vi "AlliGator Read set File.vi"(8 "Error In":errorcluster, 11 "Image Folder Path":path) -> (0 "Error Out":errorcluster, 1 "Metadata":T1 {"Date" format="%<%x %.3X>T"}, 2 "File Info String":string, 3 ".set File dup":path, 5 "File info":variant)   [LabVIEW 2021, in "AlliGator Files.lvlib"]
doc: "Tries to extract FLI dataset metadata corresponding to one of LaVision formats."
uses:
  AlliGator Files.lvlib
  AlliGator RecSettings Metadata.ctl
  AlliGator RecSettings Metadata Field.ctl
  <vilib>/Utility/error.llb/whitespace.ctl
  Time/PicoStart Date.ctl
  Strings/Strings.lvlib
  Time/Time.lvlib
panel:
  out "Time (s)":dbl
  # "see the AlliGator License on the block diagram (Ctrl+E or Window:Show Block Diagram)"
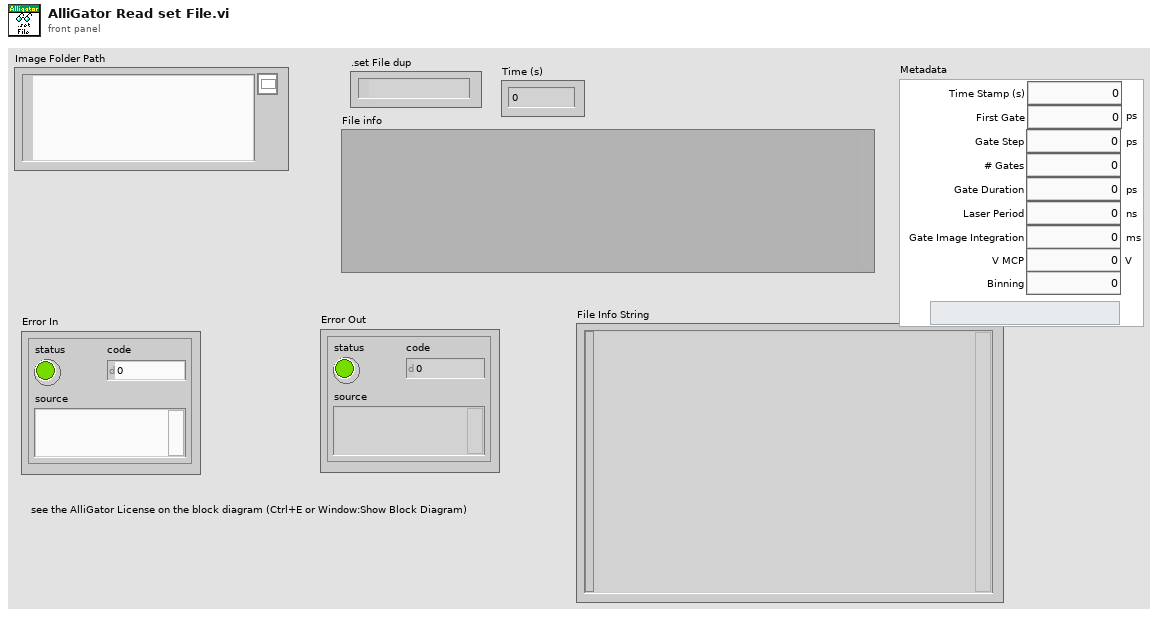
[diagram p1: front panel]
types:
  T1 = typedef "AlliGator Files.lvlib/AlliGator RecSettings Metadata.ctl" = cluster{"Time Stamp (s)":dbl, "First Gate":dbl[unit], "Gate Step":dbl[unit], "# Gates":i32, "Gate Duration":dbl[unit], "Laser Period":dbl[unit], "Gate Image Integration":dbl[unit], "Date":timestamp, "V MCP":dbl[unit], "Binning":dbl}
  T2 = typedef "AlliGator Files.lvlib/AlliGator RecSettings Metadata Field.ctl" = enum16{"Time", "Gate Start", "Gate Step", "# Gates", "Gate Duration", "Laser Period", "Gate Image Integration", "MCP Voltage", "Binning"}
  T3 = typedef "Time.lvlib/PicoStart Date.ctl" = cluster{"Day in Week":string, "Month":string, "Day":i32, "Hours":i32, "Minutes":i32, "Seconds":i32, "Year":i32}
  T4 = typedef "whitespace.ctl" = u16
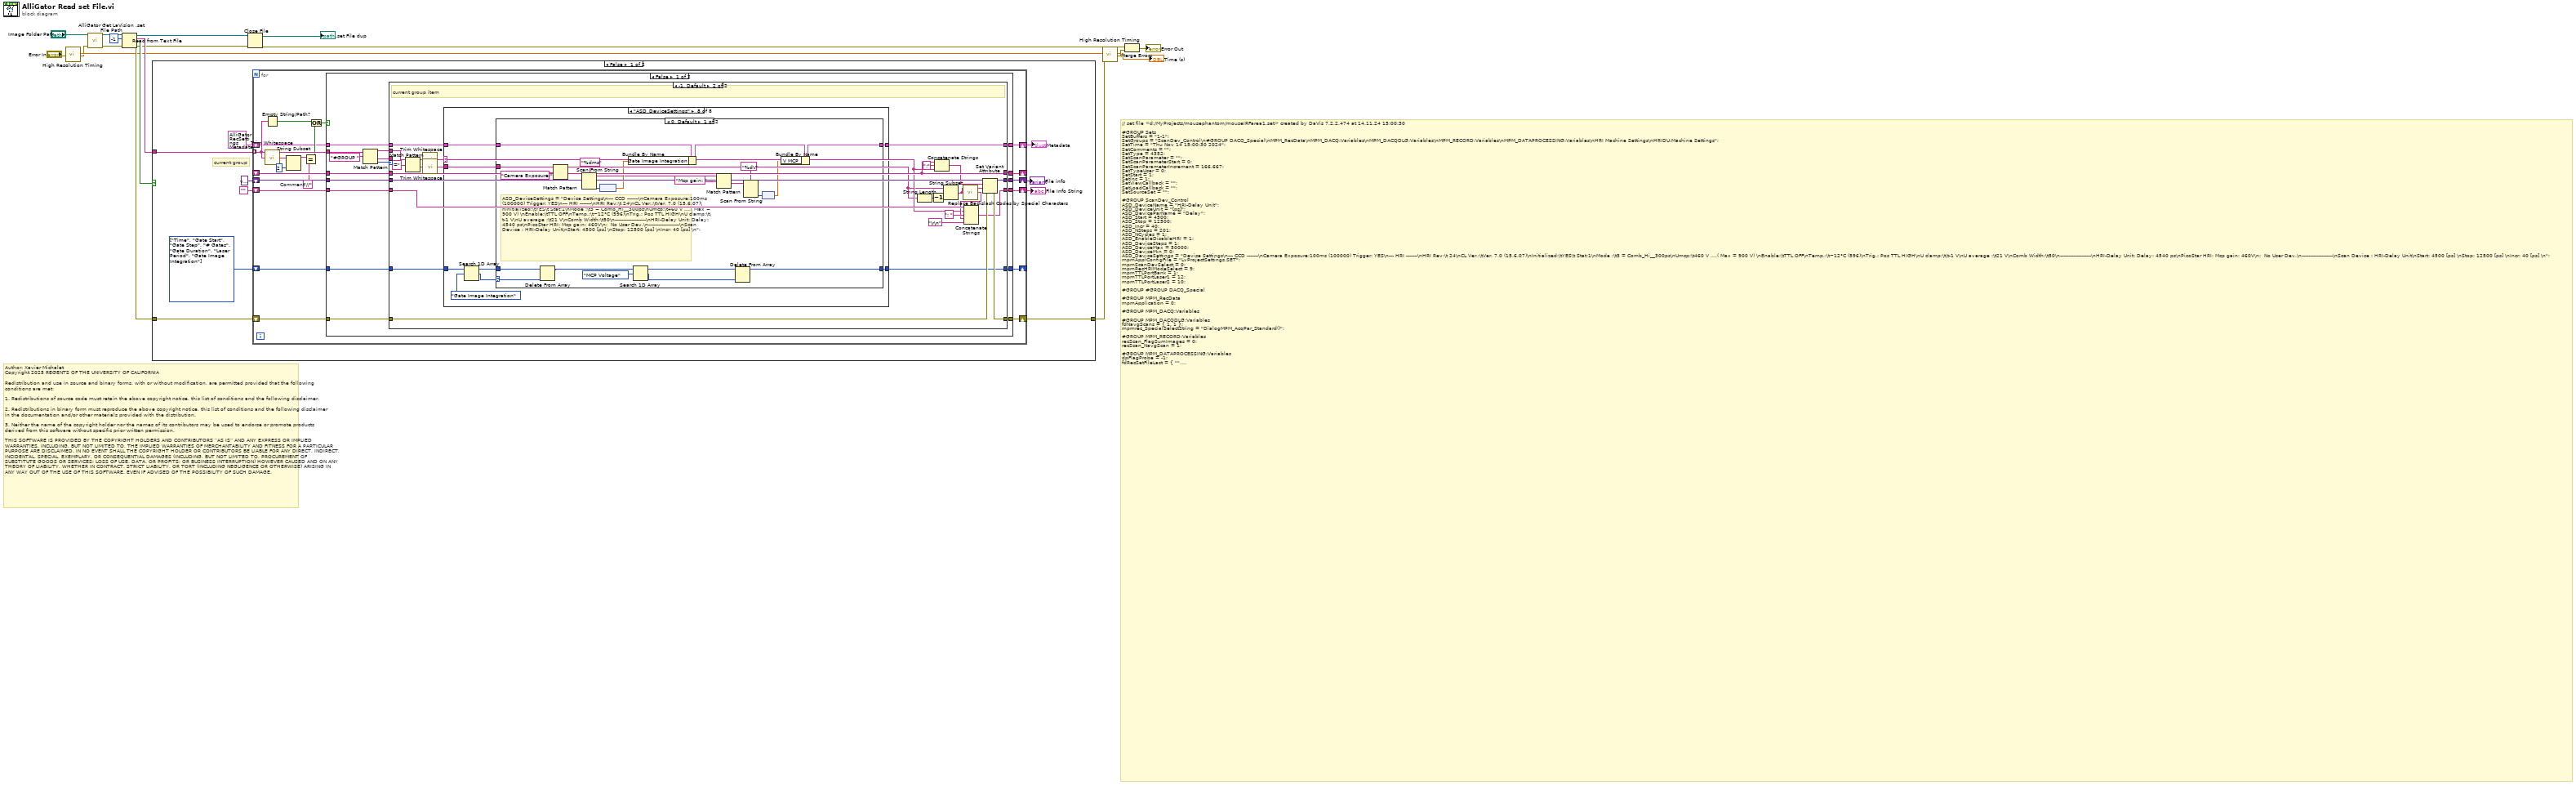
[diagram p0: block diagram]
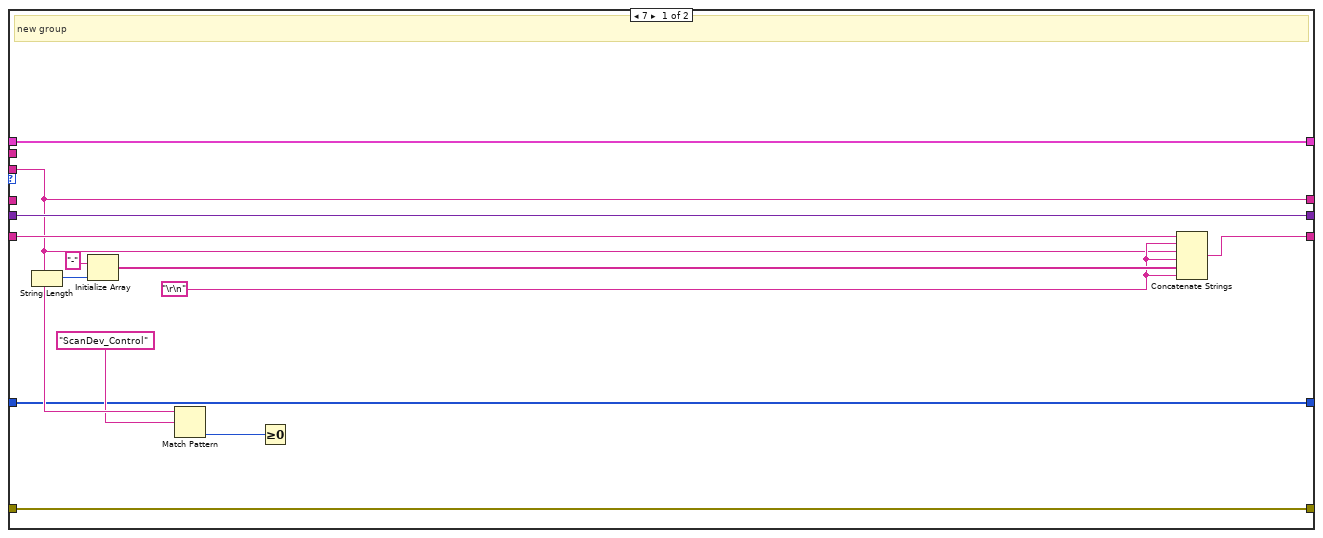
[diagram p2: hidden frame]
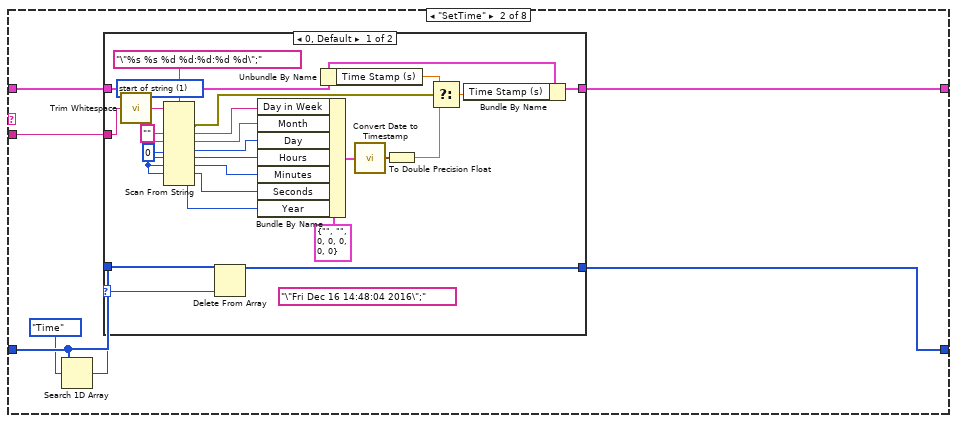
[diagram p4: hidden frame]
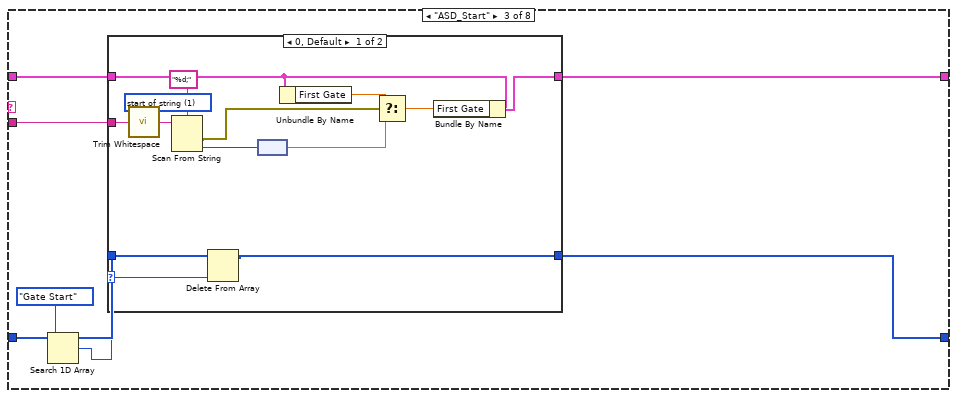
[diagram p6: hidden frame]
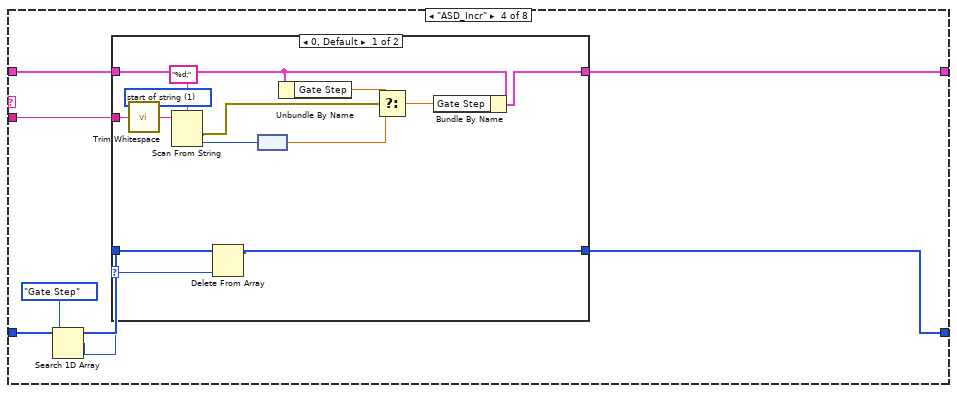
[diagram p8: hidden frame]
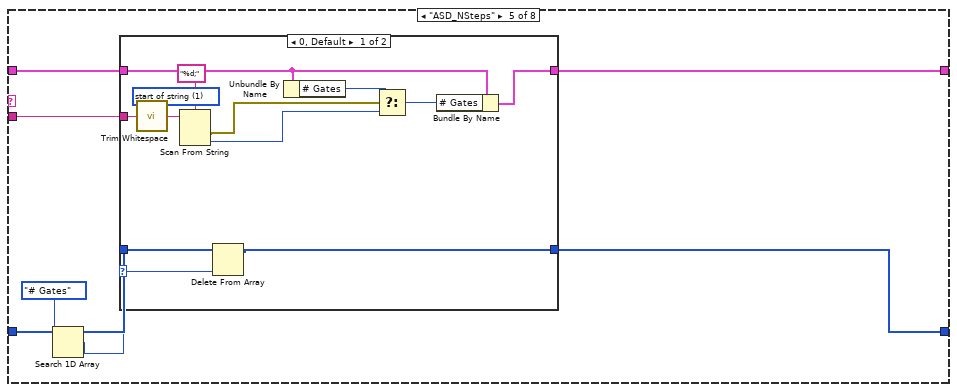
[diagram p10: hidden frame]
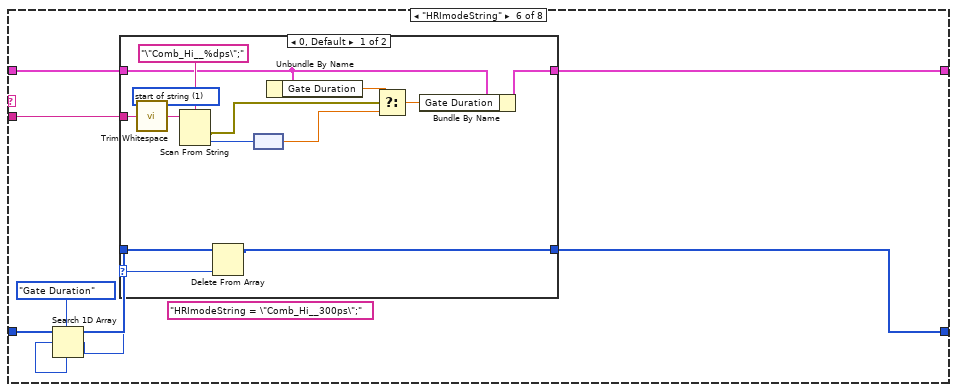
[diagram p12: hidden frame]
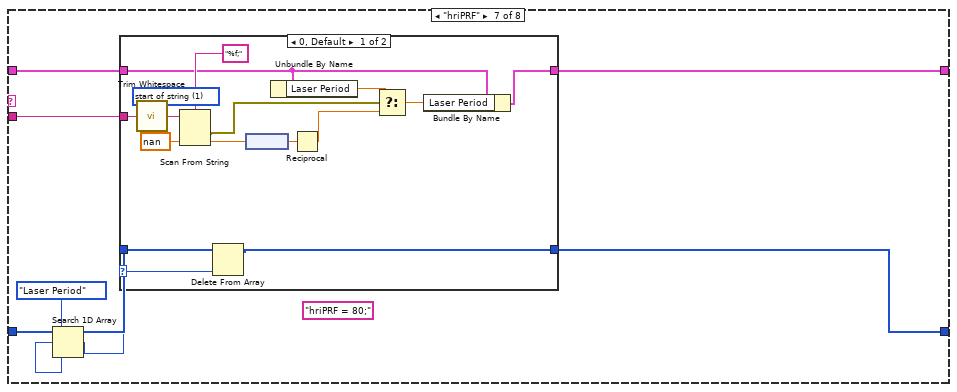
[diagram p14: hidden frame]
diagram:
  # "// set file <d:/MyProjects/mousephantom/mouseIRFarea1.set> created by DaVis 7.2.2.474 at 14.11.24 15:00:30\n\n#GROUP Sets\nSetBuffers = \"1-1\";  \nSetGroups = \"ScanDev_Control\\n#GROUP DACQ_Special\\nMPM_RecData\\nMPM_DACQ:Variables\\nMPM_DACQDLG:Variables\\nMPM_RECORD:Variables\\nMPM_DATAPROCESSING:Variables\\nHRI Machine Settings\\nHRIDU:Machine Settings\";\nSetTime = \"Thu Nov 14 15:00:30 2024\";\nSetComments = \"\";\nSetType = 4352;\nSetScanParameter = \"\";\nSetScanParameterStart = 0;\nSetScanParameterIncrement = 166.667;\nSetTypeUser = 0;\nSetStart = 1;\nSetInc = 1;\nSetViewCallback = \"\";\nSetLoadCallback = \"\";\nSetSourceSet = \"\";\n\n#GROUP ScanDev_Control\nASD_DeviceName = \"HRI-Delay Unit\";\nASD_DeviceUnit = \"[ps]\";\nASD_DeviceParName = \"Delay\";\nASD_Start = 4500;\nASD_Stop = 12500;\nASD_Incr = 40;\nASD_NSteps = 201;\nASD_NCycles = 1;\nASD_EnableDisableHRI = 1;\nASD_DeviceSteps = 1;\nASD_DeviceMax = 50000;\nASD_DeviceMin = 0;\nASD_DeviceSettings = \"Device Settings\\n--- CCD -------\\nCamera Exposure:100ms (100000) Trigger: YES\\n--- HRI -------\\nHRI Rev:\\t 24\\nCL Ver.:\\tVer. 7.0 (15.6.07)\\nInitialized:\\tYES\\t Stat:1\\nMode :\\t3 = Comb_Hi__300ps\\nUmcp:\\t460 V ....( Max = 900 V) \\nEnable:\\tTTL OFF\\nTemp.:\\t~12°C (596)\\nTrig.: Pos TTL HIGH\\nU clamp:\\t\\t-1 V\\nU average :\\t21 V\\nComb Width:\\t50\\n-------------------\\nHRI-Delay Unit: Delay: 4540 ps\\nPicoStar HRI: Mcp gain: 460V\\n:  No User Dev.\\n-------------------\\nScan Device : HRI-Delay Unit\\nStart: 4500 [ps] \\nStop: 12500 [ps] \\nIncr: 40 [ps] \\n\";\nmpmApplConfigFile = \"LvProjectSettings.SET\";\nmpmScanDevSelect = 0;\nmpmRecHRIModeSelect = 9;\nmpmTTLPortBank = 1;\nmpmTTLPortLaser1 = 12;\nmpmTTLPortLaser2 = 10;\n\n#GROUP #GROUP DACQ_Special\n\n#GROUP MPM_RecData\nmpmApplication = 0;\n\n#GROUP MPM_DACQ:Variables\n\n#GROUP MPM_DACQDLG:Variables\nfdNavgScans = { 1, 1 };\nmpmrec_SpecialSelectString = \"DialogMPM_AcqPar_Standard()\";\n\n#GROUP MPM_RECORD:Variables\nrecScan_FlagSumImages = 0;\nrecScan_NavgScan = 1;\n\n#GROUP MPM_DATAPROCESSING:Variables\ndpFlagProbe = -1;\nfdRecSetFileLast = { \"\", \"\" };\nmpmFlag_UseFitDLL = 1;\nflimfd_Freq = 80;\nflimFlagShowTrace = 1;\n\n#GROUP HRI Machine Settings\nhriPRF = 80;\nHRIType = 0;\nHRIMode = 3;\nHRIGain = 430;\nHRITrig_Edge = 1;\nHRITrig_Typ = 0;\nHRITrig_Level = 0;\nHRITrig_Term = 0;\nHRIThresh = 0.4;\nHRIClamp = -1;\nHRIAverage = 21;\nHRICombWidth = 50;\nHRIRFgain = 60;\nHRIRFgainIncr = 10;\nhriTempString = \"~12°C (596)\";\nHRIRateTune = 3;\nHRImodeString = \"Comb_Hi__300ps\";\nHRIGOIMode = 0;\n\n#GROUP HRIDU:Machine Settings\nhridu_40MHz_copy = 0;\nhridu_Trg_Coupling_copy = 1;\nhridu_Trg_Term_copy = 1;\nhridu_Trg_Edge_copy = 1;\nhridu_Trg_Attenuator_copy = 0;\nhridu_Trg_Thresh_copy = 102;\nhridu_Delay_copy = 7740;\nhridu_ScanDelayStart_copy = 0;\nhridu_ScanDelayStop_copy = 12000;\nhridu_ScanDelayIncr_copy = 40;"
  # "Author: Xavier Michalet\nCopyright 2025 REGENTS OF THE UNIVERSITY OF CALIFORNIA\n\nRedistribution and use in source and binary forms, with or without modification, are permitted provided that the following conditions are met:\n\n1. Redistributions of source code must retain the above copyright notice, this list of conditions and the following disclaimer.\n\n2. Redistributions in binary form must reproduce the above copyright notice, this list of conditions and the following disclaimer in the documentation and/or other materials provided with the distribution.\n\n3. Neither the name of the copyright holder nor the names of its contributors may be used to endorse or promote products derived from this software without specific prior written permission.\n\nTHIS SOFTWARE IS PROVIDED BY THE COPYRIGHT HOLDERS AND CONTRIBUTORS “AS IS” AND ANY EXPRESS OR IMPLIED WARRANTIES, INCLUDING, BUT NOT LIMITED TO, THE IMPLIED WARRANTIES OF MERCHANTABILITY AND FITNESS FOR A PARTICULAR PURPOSE ARE DISCLAIMED. IN NO EVENT SHALL THE COPYRIGHT HOLDER OR CONTRIBUTORS BE LIABLE FOR ANY DIRECT, INDIRECT, INCIDENTAL, SPECIAL, EXEMPLARY, OR CONSEQUENTIAL DAMAGES (INCLUDING, BUT NOT LIMITED TO, PROCUREMENT OF SUBSTITUTE GOODS OR SERVICES; LOSS OF USE, DATA, OR PROFITS; OR BUSINESS INTERRUPTION) HOWEVER CAUSED AND ON ANY THEORY OF LIABILITY, WHETHER IN CONTRACT, STRICT LIABILITY, OR TORT (INCLUDING NEGLIGENCE OR OTHERWISE) ARISING IN ANY WAY OUT OF THE USE OF THIS SOFTWARE, EVEN IF ADVISED OF THE POSSIBILITY OF SUCH DAMAGE."
  n1 = call "High Resolution Timing.vi"("Error In"="Error In") -> ("elapsed (relative) seconds"=w7:dbl, "Error Out"=w2:errorcluster)  [unwired: 16 in, 1 out]
  n2 = call "AlliGator Get LaVision .set File Path.vi"("Error In"=w2, "Gate Image Folder Path"="Image Folder Path") -> ("Error Out"=w1:errorcluster, ".set File Path"=w4:path)  [unwired: 8 in]
  n3 = Read from Text File(file (use dialog)=w4, count=-1, error in=w1) -> (refnum out=w16:refnum<file>, text=w14:string[], cancelled=w13:bool, error out=w11:errorcluster)  [unwired: 1 in]
  n4 = case shown="False" w13 {
    tunnel: w14 -> [w27 _]
    tunnel: w11 -> [w24 w291]
    tunnel: [w23 w291] -> w10
    frame False {
      w19 = T2[] [enum."Time", enum."Gate Start", enum."Gate Step", enum."# Gates", enum."Gate Duration", enum."Laser Period", enum."Gate Image Integration"] items=["Time", "Gate Start", "Gate Step", "# Gates", "Gate Duration", "Laser Period", "Gate Image Integration", "MCP Voltage", "Binning"] ("Array")
      # "current group"
      n5 = for {
        tunnel: w27 -> [w41] mode=indexing
        shift-right: [w45] -> _
        shift-left: _ -> [w46]
        shift-right: [w44] -> w25
        shift-left: variant -> [w43]
        shift-right: [w34] -> w23
        shift-left: w24 -> [w35]
        shift-right: [w32] -> w21
        shift-left: "" -> [w33]
        shift-right: [w31] -> w20
        shift-left: T1 {"Time Stamp (s)"=nan, "First Gate"=nan, "Gate Step"=nan, "# Gates"=0, "Gate Duration"=nan, "Laser Period"=nan, "Gate Image Integration"=nan, "Date"=timestamp(0 s since 1904-01-01), "V MCP"=nan, "Binning"=nan} ("Metadata") -> [w30]
        shift-right: [w28] -> _
        shift-left: w19 -> [w29]
        w37 = "//"  # Comment
        n6 = call <vilib>:"Trim Whitespace.vi"("string"=w41) -> ("trimmed string"=w40:string)  [unwired: 1 in]
        n7 = Empty String/Path?(string/path=w41) -> (empty?=w47:bool)
        n8 = String Subset(string=w40, length (rest)=2 ("length (rest)")) -> (substring=w38:string)  [unwired: 1 in]
        n9 = Equal?(x=w38, y=w37) -> (x = y?=w36:bool)
        n10 = Or(x=w47, y=w36) -> (x .or. y?=w42:bool)
        n11 = case shown="False" w42 {
          tunnel: w41 -> [w63 _]
          tunnel: w46 -> [w57 w290]
          tunnel: [w60 w290] -> w45
          tunnel: [w59 w289] -> w44
          tunnel: w43 -> [w58 w289]
          tunnel: w35 -> [w55 w288]
          tunnel: [w54 w288] -> w34
          tunnel: w33 -> [w53 w287]
          tunnel: [w52 w287] -> w32
          tunnel: [w51 w286] -> w31
          tunnel: w30 -> [w50 w286]
          tunnel: w29 -> [w49 w285]
          tunnel: [w48 w285] -> w28
          frame False {
            n12 = Match Pattern(string=w63, regular expression="#GROUP ") -> (before substring=w56:string, after substring=w61:string, offset past match=w62:i32)  [unwired: 1 in, 1 out]
            n13 = case shown="-1, Default" w62 {
              tunnel: w61 -> [w68 _]
              tunnel: [w68 w96] -> w60
              tunnel: [w77 w100] -> w59
              tunnel: w58 -> [w77 w99]
              tunnel: w57 -> [_ w96]
              tunnel: w56 -> [_ w94]
              tunnel: w55 -> [w76 w93]
              tunnel: [w76 w92] -> w54
              tunnel: w53 -> [w75 w91]
              tunnel: [w71 w87] -> w52
              tunnel: [w69 w81] -> w51
              tunnel: w50 -> [w69 w80]
              tunnel: w49 -> [w65 w79]
              tunnel: [w65 w78] -> w48
              frame 7 {
                w70 = "\r\n"
                # "new group"
                n14 = String Length(string=w68) -> (length=w74:i32)
                n15 = Initialize Array("-", w74) -> (w72:string[])
                n16 = Match Pattern(string=w68, regular expression="ScanDev_Control") -> (offset past match=w66:i32)  [unwired: 1 in, 3 out]
                n17 = Greater Or Equal To 0?(x=w66) -> ()  [unwired: 1 out]
                n18 = Concatenate Strings(w75, w70, w68, w70, w72, w70) -> (w71:string)
              }
              frame -1, Default {
                # "current group item"
                n19 = Match Pattern(string=w94, regular expression="=") -> (before substring=w101:string, after substring=w83:string)  [unwired: 1 in, 2 out]
                n20 = call <vilib>:"Trim Whitespace.vi"("string"=w101) -> ("trimmed string"=w84:string)  [unwired: 1 in]
                n21 = call <vilib>:"Trim Whitespace.vi"("string"=w83) -> ("trimmed string"=w82:string)  [unwired: 1 in]
                n22 = case shown="\"ASD_DeviceSettings\"" w84 {
                  tunnel: w82 -> [_ w111 w144 w167 w190 w212 w235 w260]
                  tunnel: [w104 w109 w145 w168 w191 w213 w236 w261] -> w81
                  tunnel: w80 -> [w104 w110 w143 w166 w189 w211 w234 w259]
                  tunnel: w79 -> [w103 w107 w141 w164 w187 w209 w232 w257]
                  tunnel: [w103 w108 w139 w162 w185 w207 w230 w255] -> w78
                  frame "", Default {
                  }
                  frame "SetTime" {
                    n23 = Search 1D Array(1D array=w107, element=AlliGator_RecSettings_Metadata_Field."Time" ("Metadata Field")) -> (index of element=w105:i32)  [unwired: 1 in]
                    n24 = case shown="0, Default" w105 {
                      selector: w105 -> [w112 _]
                      tunnel: w111 -> [w117 _]
                      tunnel: w110 -> [w116 w138]
                      tunnel: [w115 w138] -> w109
                      tunnel: [w114 w137] -> w108
                      tunnel: w107 -> [w113 w137]
                      frame 0, Default {
                        (unwired) "\"Fri Dec 16 14:48:04 2016\";"
                        w123 = 0 ("default value 3")
                        w124 = "" ("default value 1")
                        w135 = T4 1 items=["both", "start of string", "end of string"] ("location (both)")
                        n25 = call <vilib>:"Trim Whitespace.vi"("string"=w117, "location (both)"=w135) -> ("trimmed string"=w126:string)
                        n26 = Scan From String(format string="\"%s %s %d %d:%d:%d %d\";", input string=w126, default 1=w124, default 2=w124, default 3=w123, default 4=w123, default 5=w123, default 6=w123) -> (error out=w122:errorcluster, output 1=w134:string, output 2=w133:string, output 3=w132:i32, output 4=w131:i32, output 5=w130:i32, output 6=w129:i32, output 7=w118:i32)  [unwired: 3 in, 2 out]
                        n27 = Delete From Array(array=w113, index=w112) -> (array with subset deleted=w114:T2[])  [unwired: 1 in, 1 out]
                        n28 = Bundle By Name(cluster=T3 {"Day in Week"="", "Month"="", "Day"=0, "Hours"=0, "Minutes"=0, "Seconds"=0, "Year"=0}, "Day in Week"=w134, "Month"=w133, "Day"=w132, "Hours"=w131, "Minutes"=w130, "Seconds"=w129, "Year"=w118) -> (w128:T3)
                        n29 = Unbundle By Name(w116) -> ("Time Stamp (s)"=w119:dbl)
                        n30 = call "Convert Date to Timestamp.vi"("Date"=w128) -> ("Time Stamp"=w136:timestamp)  [unwired: 8 in]
                        n31 = To Double Precision Float(number=w136) -> (double precision float=w120:dbl)
                        n32 = Select(t=w119, s=w122, f=w120) -> (s? t:f=w121:dbl)
                        n33 = Bundle By Name(cluster=w116, "Time Stamp (s)"=w121) -> (w115:T1)
                      }
                      frame -1 {
                      }
                    }
                  }
                  frame "ASD_Start" {
                    n34 = Search 1D Array(1D array=w141, element=AlliGator_RecSettings_Metadata_Field."Gate Start" ("Metadata Field")) -> (index of element=w140:i32)  [unwired: 1 in]
                    n35 = case shown="0, Default" w140 {
                      selector: w140 -> [w147 _]
                      tunnel: [w159 w161] -> w145
                      tunnel: w144 -> [w155 _]
                      tunnel: w143 -> [w152 w161]
                      tunnel: w141 -> [w148 w160]
                      tunnel: [w146 w160] -> w139
                      frame 0, Default {
                        w158 = T4 1 items=["both", "start of string", "end of string"] ("location (both)")
                        n36 = call <vilib>:"Trim Whitespace.vi"("string"=w155, "location (both)"=w158) -> ("trimmed string"=w157:string)
                        n37 = Scan From String(format string="%d;", input string=w157) -> (error out=w154:errorcluster, output 1=w150:i32)  [unwired: 3 in, 2 out]
                        n38 = Delete From Array(array=w148, index=w147) -> (array with subset deleted=w146:T2[])  [unwired: 1 in, 1 out]
                        n39 = node(w150) -> (w149:dbl[unit])
                        n40 = Unbundle By Name(w152) -> ("First Gate"=w151:dbl[unit])
                        n41 = Select(t=w151, s=w154, f=w149) -> (s? t:f=w153:dbl[unit])
                        n42 = Bundle By Name(cluster=w152, "First Gate"=w153) -> (w159:T1)
                      }
                      frame -1 {
                      }
                    }
                  }
                  frame "ASD_Incr" {
                    n43 = Search 1D Array(1D array=w164, element=AlliGator_RecSettings_Metadata_Field."Gate Step" ("Metadata Field")) -> (index of element=w163:i32)  [unwired: 1 in]
                    n44 = case shown="0, Default" w163 {
                      selector: w163 -> [w170 _]
                      tunnel: [w182 w184] -> w168
                      tunnel: w167 -> [w178 _]
                      tunnel: w166 -> [w175 w184]
                      tunnel: w164 -> [w171 w183]
                      tunnel: [w169 w183] -> w162
                      frame 0, Default {
                        w181 = T4 1 items=["both", "start of string", "end of string"] ("location (both)")
                        n45 = call <vilib>:"Trim Whitespace.vi"("string"=w178, "location (both)"=w181) -> ("trimmed string"=w180:string)
                        n46 = Scan From String(format string="%d;", input string=w180) -> (error out=w177:errorcluster, output 1=w173:i32)  [unwired: 3 in, 2 out]
                        n47 = Delete From Array(array=w171, index=w170) -> (array with subset deleted=w169:T2[])  [unwired: 1 in, 1 out]
                        n48 = node(w173) -> (w172:dbl[unit])
                        n49 = Unbundle By Name(w175) -> ("Gate Step"=w174:dbl[unit])
                        n50 = Select(t=w174, s=w177, f=w172) -> (s? t:f=w176:dbl[unit])
                        n51 = Bundle By Name(cluster=w175, "Gate Step"=w176) -> (w182:T1)
                      }
                      frame -1 {
                      }
                    }
                  }
                  frame "ASD_NSteps" {
                    n52 = Search 1D Array(1D array=w187, element=AlliGator_RecSettings_Metadata_Field."# Gates" ("Metadata Field")) -> (index of element=w186:i32)  [unwired: 1 in]
                    n53 = case shown="0, Default" w186 {
                      selector: w186 -> [w193 _]
                      tunnel: [w204 w206] -> w191
                      tunnel: w190 -> [w200 _]
                      tunnel: w189 -> [w197 w206]
                      tunnel: w187 -> [w194 w205]
                      tunnel: [w192 w205] -> w185
                      frame 0, Default {
                        w203 = T4 1 items=["both", "start of string", "end of string"] ("location (both)")
                        n54 = call <vilib>:"Trim Whitespace.vi"("string"=w200, "location (both)"=w203) -> ("trimmed string"=w202:string)
                        n55 = Scan From String(format string="%d;", input string=w202) -> (error out=w199:errorcluster, output 1=w195:i32)  [unwired: 3 in, 2 out]
                        n56 = Delete From Array(array=w194, index=w193) -> (array with subset deleted=w192:T2[])  [unwired: 1 in, 1 out]
                        n57 = Unbundle By Name(w197) -> ("# Gates"=w196:i32)
                        n58 = Select(t=w196, s=w199, f=w195) -> (s? t:f=w198:i32)
                        n59 = Bundle By Name(cluster=w197, "# Gates"=w198) -> (w204:T1)
                      }
                      frame -1 {
                      }
                    }
                  }
                  frame "HRImodeString" {
                    (unwired) "HRImodeString = \"Comb_Hi__300ps\";" ("string")
                    n60 = Search 1D Array(1D array=w209, element=AlliGator_RecSettings_Metadata_Field."Gate Duration" ("Metadata Field")) -> (index of element=w208:i32)  [unwired: 1 in]
                    n61 = case shown="0, Default" w208 {
                      selector: w208 -> [w216 _]
                      tunnel: [w227 w229] -> w213
                      tunnel: w212 -> [w223 _]
                      tunnel: w211 -> [w220 w229]
                      tunnel: w209 -> [w217 w228]
                      tunnel: [w215 w228] -> w207
                      frame 0, Default {
                        w226 = T4 1 items=["both", "start of string", "end of string"] ("location (both)")
                        n62 = call <vilib>:"Trim Whitespace.vi"("string"=w223, "location (both)"=w226) -> ("trimmed string"=w225:string)
                        n63 = Scan From String(format string="\"Comb_Hi__%dps\";", input string=w225) -> (error out=w222:errorcluster, output 1=w218:i32)  [unwired: 3 in, 2 out]
                        n64 = Delete From Array(array=w217, index=w216) -> (array with subset deleted=w215:T2[])  [unwired: 1 in, 1 out]
                        n65 = node(w218) -> (w214:dbl[unit])
                        n66 = Unbundle By Name(w220) -> ("Gate Duration"=w219:dbl[unit])
                        n67 = Select(t=w219, s=w222, f=w214) -> (s? t:f=w221:dbl[unit])
                        n68 = Bundle By Name(cluster=w220, "Gate Duration"=w221) -> (w227:T1)
                      }
                      frame -1 {
                      }
                    }
                  }
                  frame "hriPRF" {
                    (unwired) "hriPRF = 80;" ("string")
                    n69 = Search 1D Array(1D array=w232, element=AlliGator_RecSettings_Metadata_Field."Laser Period" ("Metadata Field")) -> (index of element=w231:i32)  [unwired: 1 in]
                    n70 = case shown="0, Default" w231 {
                      selector: w231 -> [w241 _]
                      tunnel: [w252 w254] -> w236
                      tunnel: w235 -> [w248 _]
                      tunnel: w234 -> [w245 w254]
                      tunnel: w232 -> [w242 w253]
                      tunnel: [w240 w253] -> w230
                      frame 0, Default {
                        w251 = T4 1 items=["both", "start of string", "end of string"] ("location (both)")
                        n71 = call <vilib>:"Trim Whitespace.vi"("string"=w248, "location (both)"=w251) -> ("trimmed string"=w250:string)
                        n72 = Scan From String(format string="%f;", input string=w250, default 1=nan ("default value 1")) -> (error out=w247:errorcluster, output 1=w243:dbl)  [unwired: 2 in, 2 out]
                        n73 = Delete From Array(array=w242, index=w241) -> (array with subset deleted=w240:T2[])  [unwired: 1 in, 1 out]
                        n74 = node(w243) -> (w239:dbl[unit])
                        n75 = Unbundle By Name(w245) -> ("Laser Period"=w244:dbl[unit])
                        n76 = Reciprocal(x=w239) -> (1/x=w238:dbl[unit])
                        n77 = Select(t=w244, s=w247, f=w238) -> (s? t:f=w246:dbl[unit])
                        n78 = Bundle By Name(cluster=w245, "Laser Period"=w246) -> (w252:T1)
                      }
                      frame -1 {
                      }
                    }
                  }
                  frame "ASD_DeviceSettings" {
                    n79 = Search 1D Array(1D array=w257, element=AlliGator_RecSettings_Metadata_Field."Gate Image Integration" ("Metadata Field")) -> (index of element=w256:i32)  [unwired: 1 in]
                    n80 = case shown="0, Default" w256 {
                      selector: w256 -> [w280 _]
                      tunnel: [w268 w284] -> w261
                      tunnel: w260 -> [w274 _]
                      tunnel: w259 -> [w282 w284]
                      tunnel: w257 -> [w281 w283]
                      tunnel: [w265 w283] -> w255
                      frame 0, Default {
                        # "ASD_DeviceSettings = \"Device Settings\\n--- CCD -------\\nCamera Exposure:100ms (100000) Trigger: YES\\n--- HRI -------\\nHRI Rev:\\t 24\\nCL Ver.:\\tVer. 7.0 (15.6.07)\\nInitialized:\\tYES\\t Stat:1\\nMode :\\t3 = Comb_Hi__300ps\\nUmcp:\\t460 V ....( Max = 900 V) \\nEnable:\\tTTL OFF\\nTemp.:\\t~12°C (596)\\nTrig.: Pos TTL HIGH\\nU clamp:\\t\\t-1 V\\nU average :\\t21 V\\nComb Width:\\t50\\n-------------------\\nHRI-Delay Unit: Delay: 4540 ps\\nPicoStar HRI: Mcp gain: 460V\\n:  No User Dev.\\n-------------------\\nScan Device : HRI-Delay Unit\\nStart: 4500 [ps] \\nStop: 12500 [ps] \\nIncr: 40 [ps] \\n\";"
                        n81 = Delete From Array(array=w281, index=w280) -> (array with subset deleted=w264:T2[])  [unwired: 1 in, 1 out]
                        n82 = Match Pattern(string=w274, regular expression="Camera Exposure:") -> (after substring=w278:string)  [unwired: 1 in, 3 out]
                        n83 = Scan From String(format string="%dms", input string=w278) -> (remaining string=w273:string, output 1=w276:i32)  [unwired: 3 in, 2 out]
                        n84 = node(w276) -> (w275:dbl[unit])
                        n85 = Bundle By Name(cluster=w282, "Gate Image Integration"=w275) -> (w269:T1)
                        n86 = Search 1D Array(1D array=w264, element=AlliGator_RecSettings_Metadata_Field."MCP Voltage") -> (index of element=w262:i32)  [unwired: 1 in]
                        n87 = Match Pattern(string=w273, regular expression="Mcp gain: ") -> (after substring=w271:string)  [unwired: 1 in, 3 out]
                        n88 = Delete From Array(array=w264, index=w262) -> (array with subset deleted=w265:T2[])  [unwired: 1 in, 1 out]
                        n89 = Scan From String(format string="%dV", input string=w271) -> (output 1=w267:i32)  [unwired: 3 in, 3 out]
                        n90 = node(w267) -> (w266:dbl[unit])
                        n91 = Bundle By Name(cluster=w269, "V MCP"=w266) -> (w268:T1)
                      }
                      frame -1 {
                      }
                    }
                  }
                }
                n92 = String Length(string=w82) -> (length=w98:i32)
                n93 = Decrement(x=w98) -> (x-1=w97:i32)
                n94 = Concatenate Strings(w96, ":" ("string"), w84) -> (w90:string)
                n95 = String Subset(string=w82, length (rest)=w97) -> (substring=w88:string)  [unwired: 1 in]
                n96 = call "Replace Backslash Codes by Special Characters.vi"("String (\\n)"=w88) -> ("String (\\\\n)"=w85:string)  [unwired: 8 in]
                n97 = Concatenate Strings(w91, w84, ": " ("string"), w85, "\r\n") -> (w87:string)
                n98 = Set Variant Attribute(Variant=w99, name=w90, value=w88, error in=w93) -> (Variant out=w100:variant, error out=w92:errorcluster)  [unwired: 1 out]
              }
            }
          }
          frame True {
            # "empty line or comment"
          }
        }
      }
      "File info" <- w25
      "File Info String" <- w21
      "Metadata" <- w20
    }
    frame True {
    }
  }
  n99 = Close File(refnum=w16, error in=w11) -> (path=→".set File dup":path, error out=w15:errorcluster)
  n100 = call "High Resolution Timing.vi"("relative seconds (NaN)"=w7, "Error In"=w10) -> ("elapsed (relative) seconds"=→"Time (s)":dbl, "Error Out"=w8:errorcluster)  [unwired: 15 in, 1 out]
  n101 = Merge Errors(w15, w8) -> (→"Error Out":errorcluster)
